vi "Write Current Strings And Values [].vi"(8 "error in (no error)":errorcluster, 10 "Strings And Values []":T1, 11 "Generic Power Analyzer in":refnum<class "Generic Power Analyzer.lvclass">) -> (0 "error out":errorcluster, 3 "Generic Power Analyzer out":refnum<class "Generic Power Analyzer.lvclass">)   [LabVIEW 2016, in "Generic Power Analyzer.lvlib" / "Generic Power Analyzer.lvclass"]
uses:
  Generic Power Analyzer.lvclass
  <vilib>/Utility/miscctls.llb/LVStringsAndValuesArrayTypeDef_U16.ctl
  Generic Power Analyzer.lvclass/Generic Power Analyzer.ctl
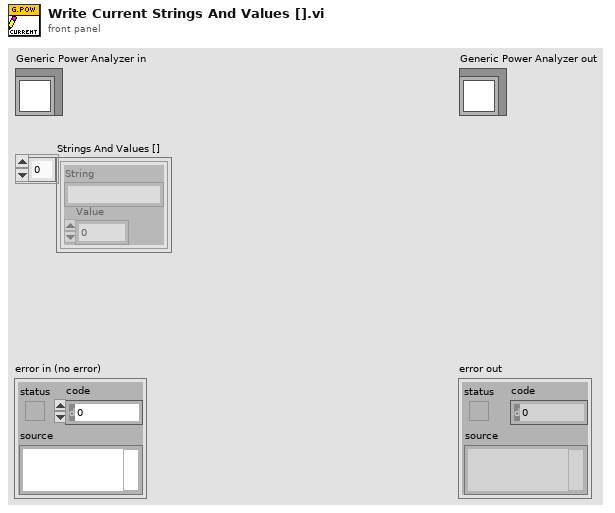
[diagram p1: front panel]
types:
  T1 = typedef "LVStringsAndValuesArrayTypeDef_U16.ctl" = cluster{"String":string, "Value":u16}[]
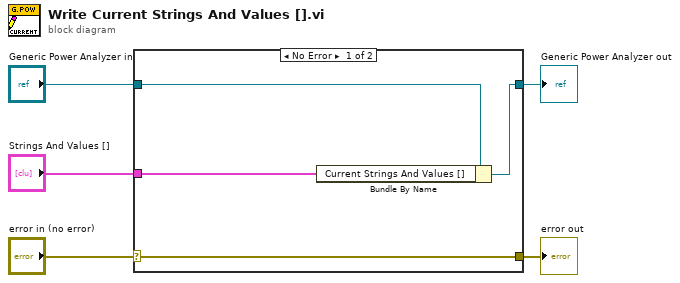
[diagram p0: block diagram]
diagram:
  n1 = case shown="No Error" "error in (no error)" {
    selector: "error in (no error)" -> [w9 w10]
    tunnel: [w9 w10] -> w4
    tunnel: [w7 w11] -> w2
    tunnel: "Generic Power Analyzer in" -> [w8 w11]
    tunnel: "Strings And Values []" -> [w6 _]
    frame No Error {
      n2 = Bundle By Name(cluster=w8, "Current Strings And Values []"=w6) -> (w7:refnum<class "Generic Power Analyzer.lvclass">)
    }
    frame Error {
    }
  }
  "error out" <- w4
  "Generic Power Analyzer out" <- w2
